vi "FGVImageArrayAux.vi"(7 "Enum":T1, 8 "error in":errorcluster, 9 "imageArrayIn":dbl[][][][](array[numeric])) -> (0 "error out":errorcluster, 1 "imageArrayOut":dbl[][][][](array[numeric]))   [LabVIEW 2016]
uses:
  controls/Enum.ctl
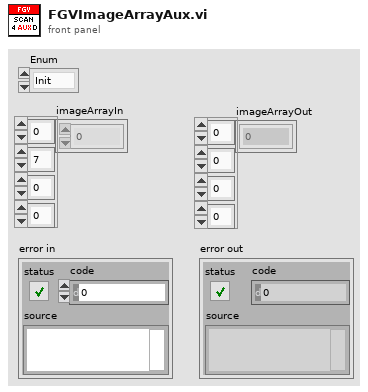
[diagram p1: front panel]
types:
  T1 = typedef "Enum.ctl" = enum16{"Init", "Read", "Write"}
  T2 = cluster{"Width":dbl, "Height":dbl, "X Offset":dbl, "Y Offset":dbl, "Angle":dbl, "Pixels/Line":u16, "Lines":u16, "Time/Line":dbl, "Scan Rate":dbl}
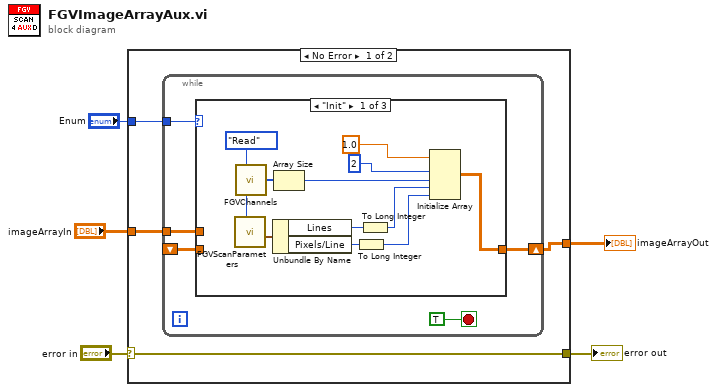
[diagram p0: block diagram]
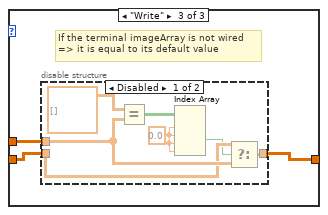
[diagram p3: hidden frame]
diagram:
  n1 = case shown="No Error" "error in" {
    selector: "error in" -> [w8 w39]
    tunnel: "Enum" -> [w9 _]
    tunnel: [w8 w39] -> w4
    tunnel: "imageArrayIn" -> [w7 w38]
    tunnel: [w6 w38] -> w1
    frame No Error {
      n2 = while {
        tunnel: w9 -> [w13]
        tunnel: w7 -> [w12]
        shift-right: [w11] -> w6
        shift-left: _ -> [w10]
        stop <- TRUE stop-if-true
        n3 = case shown="\"Init\"" w13 {
          tunnel: w12 -> [_ _ w28]
          tunnel: [w24 w26 w29] -> w11
          tunnel: w10 -> [_ w26 w27]
          frame "Init" {
            w18 = Enum."Read" ("Enum")
            n4 = call "FGVScanParameters.vi"("Enum"=w18) -> ("Scan Parameters Out"=w23:T2)  [unwired: 9 in, 1 out]
            n5 = call "FGVChannels.vi"("Enum"=w18) -> ("channelsToSaveOut"=w17:u8[])  [unwired: 6 in, 4 out]
            n6 = Unbundle By Name(w23) -> ("Lines"=w22:u16, "Pixels/Line"=w21:u16)
            n7 = Array Size(array=w17) -> (size(s)=w20:i32)
            n8 = To Long Integer(number=w21) -> (32bit integer=w15:i32)
            n9 = To Long Integer(number=w22) -> (32bit integer=w16:i32)
            n10 = Initialize Array(1.0, u8 2 ("dimension size"), w20, w16, w15) -> (w24:dbl[][][][])
          }
          frame "Read", Default {
          }
          frame "Write" {
            # "If the terminal imageArray is not wired\n=> it is equal to its default value"
            n11 = disable-structure shown="Disabled" {
              disable-tunnel: [w36 w37] -> w29
              disable-tunnel: w28 -> [w32 w37]
              disable-tunnel: w27 -> [w31 _]
              frame Disabled {
                w34 = 0.0 ("index (vol)")
                n12 = Equal?(x=dbl[][][][] [] ("imageArrayIn"), y=w32) -> (x = y?=w33:bool[][][][])
                n13 = Index Array(array=w33, index (dim 0)=w34, index (dim 1)=w34, index (dim 2)=w34, index (dim 3)=w34) -> (element=w30:bool)
                n14 = Select(t=w31, s=w30, f=w32) -> (s? t:f=w36:dbl[][][][])
              }
              frame Enabled {
              }
            }
          }
        }
      }
    }
    frame Error {
    }
  }
  "error out" <- w4
  "imageArrayOut" <- w1
